vi "while loop.vi"() -> ()   [LabVIEW 2020]
panel:
  in  "y 2":dbl
  in  "x 2":dbl
  out "x+y 2":dbl
  in  "stop 2":bool
  in  "stop":bool
  out "x+y":dbl
  in  "x":dbl
  in  "y":dbl
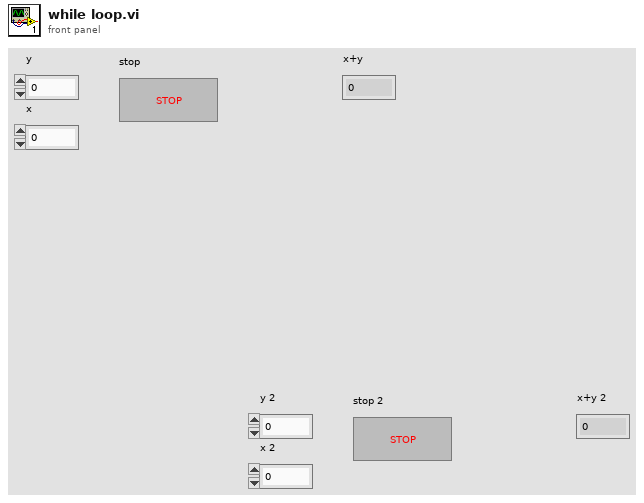
[diagram p1: front panel]
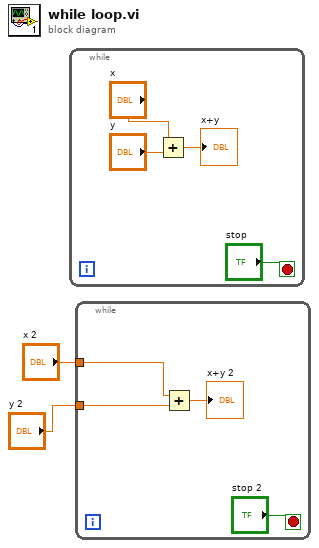
[diagram p0: block diagram]
diagram:
  n1 = while {
    stop <- "stop" stop-if-true
    n2 = Add(x="x", y="y") -> (x+y=→"x+y":dbl)
  }
  n3 = while {
    tunnel: "x 2" -> [w8]
    tunnel: "y 2" -> [w7]
    stop <- "stop 2" stop-if-true
    n4 = Add(x=w8, y=w7) -> (x+y=→"x+y 2":dbl)
  }
